vi "Update UI.vi"(0 "DAQ Controller in":refnum<class "DAQ Controller.lvclass">, 5 "QPD Voltage X":dbl format="%#_13g", 7 "QPD Voltage Y":dbl format="%#_13g", 9 "QPD  Sum":dbl format="%#_13g", 11 "error in (no error)":errorcluster) -> (4 "DAQ Controller out":refnum<class "DAQ Controller.lvclass">, 15 "error out":errorcluster)   [LabVIEW 2020, in "DAQ.lvlib" / "DAQ Controller.lvlib" / "DAQ Controller.lvclass"]
uses:
  DAQ Controller.lvclass
  DAQ Controller.lvclass/DAQ Controller.ctl
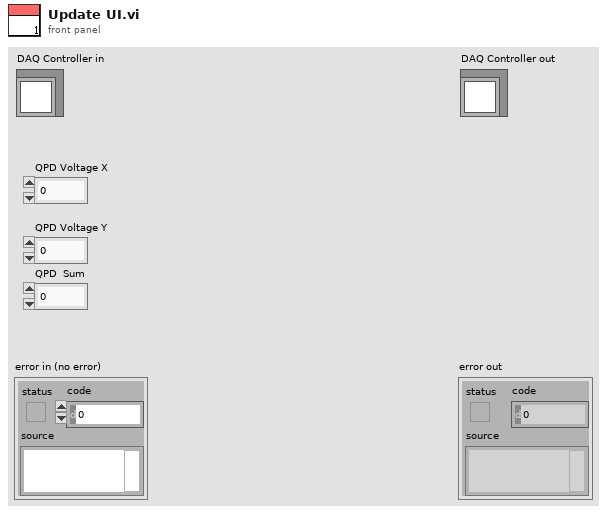
[diagram p1: front panel]
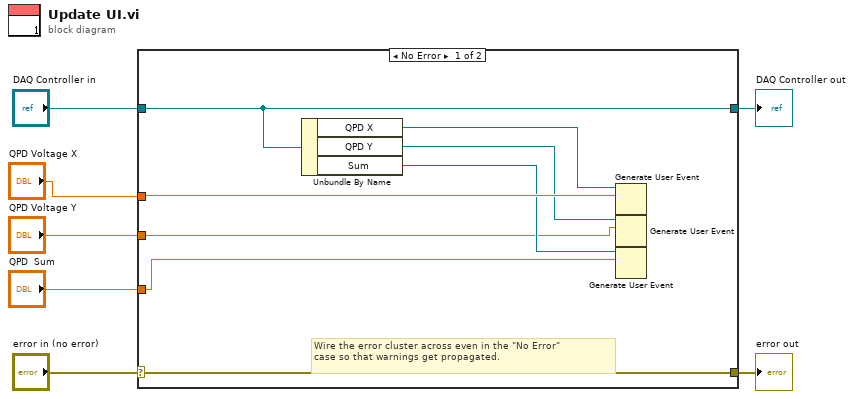
[diagram p0: block diagram]
diagram:
  n1 = case shown="No Error" "error in (no error)" {
    selector: "error in (no error)" -> [w15 w17]
    tunnel: [w15 w17] -> w6
    tunnel: [w14 w16] -> w4
    tunnel: "DAQ Controller in" -> [w14 w16]
    tunnel: "QPD Voltage X" -> [w12 _]
    tunnel: "QPD Voltage Y" -> [w9 _]
    tunnel: "QPD  Sum" -> [w8 _]
    frame No Error {
      # "Wire the error cluster across even in the \"No Error\"\ncase so that warnings get propagated."
      n2 = Unbundle By Name(w14) -> ("QPD X"=w13:refnum<user-event>, "QPD Y"=w11:refnum<user-event>, "Sum"=w10:refnum<user-event>)
      n3 = Generate User Event(user event=w13, event data cluster=w12) -> ()  [unwired: 2 in, 2 out]
      n4 = Generate User Event(user event=w11, event data cluster=w9) -> ()  [unwired: 2 in, 2 out]
      n5 = Generate User Event(user event=w10, event data cluster=w8) -> ()  [unwired: 2 in, 2 out]
    }
    frame Error {
    }
  }
  "error out" <- w6
  "DAQ Controller out" <- w4
